vi "Collapse Patterns SLM.vi"(2 "Action":u16(ring) items=["Read", "Initialize"], 7 "collapsed mode array":dbl[][](array[numeric]), 9 "Vortex":dbl[][](array[numeric]), 11 "Top hat":dbl[][](array[numeric])) -> (8 "collapsed patterns":dbl[][](array[numeric]))   [LabVIEW 2014]
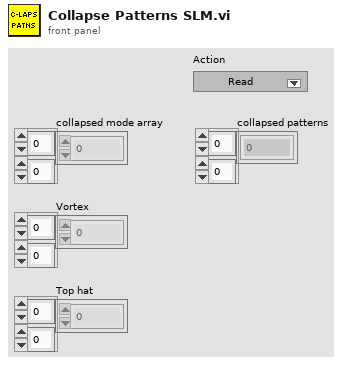
[diagram p1: front panel]
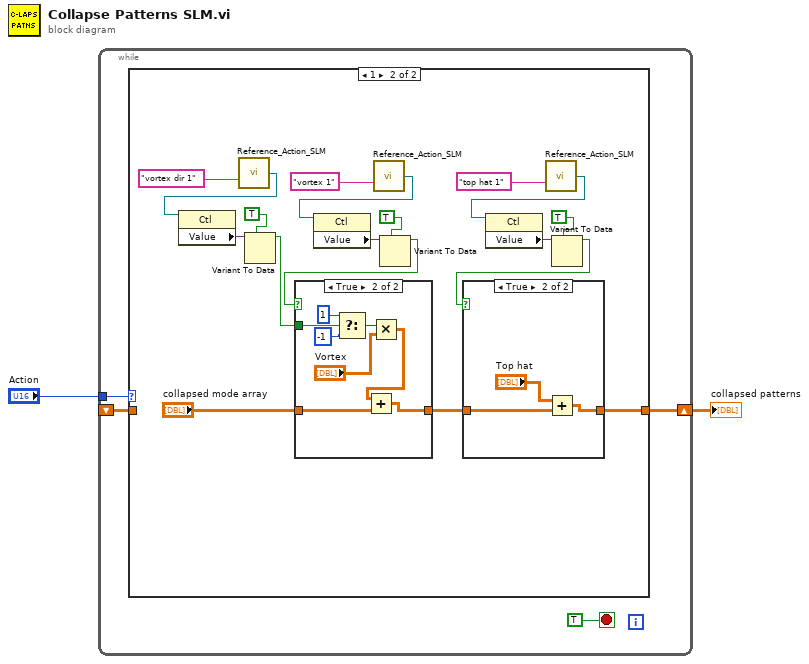
[diagram p0: block diagram]
diagram:
  n1 = while {
    shift-right: [w3] -> w1
    shift-left: _ -> [w4]
    tunnel: "Action" -> [w5]
    stop <- TRUE stop-if-true
    n2 = case shown="1" w5 {
      tunnel: w4 -> [w7 _]
      tunnel: [w7 w14] -> w3
      frame 0, Default {
      }
      frame 1 {
        n3 = call "Reference_Action_SLM.vi"("Control Name"="vortex dir 1") -> ("Ref OUT"=w9:refnum<vi>)  [unwired: 12 in, 2 out]
        n4 = property class="Ctl"(reference=w9) -> ("Value"=w11:variant)  [unwired: 1 in, 2 out]
        n5 = Variant To Data(type=TRUE, Variant=w11) -> (data=w8:bool)  [unwired: 1 in, 1 out]
        n6 = call "Reference_Action_SLM.vi"("Control Name"="vortex 1") -> ("Ref OUT"=w24:refnum<vi>)  [unwired: 12 in, 2 out]
        n7 = property class="Ctl"(reference=w24) -> ("Value"=w23:variant)  [unwired: 1 in, 2 out]
        n8 = Variant To Data(type=TRUE, Variant=w23) -> (data=w21:bool)  [unwired: 1 in, 1 out]
        n9 = case shown="True" w21 {
          tunnel: "collapsed mode array" -> [w30 w38]
          tunnel: [w30 w37] -> w15
          tunnel: w8 -> [_ w31]
          frame False {
          }
          frame True {
            n10 = Select(t=1, s=w31, f=-1) -> (s? t:f=w34:i32)
            n11 = Multiply(x=w34, y="Vortex") -> (x*y=w32:dbl[][])
            n12 = Add(x=w32, y=w38) -> (x+y=w37:dbl[][])
          }
        }
        n13 = call "Reference_Action_SLM.vi"("Control Name"="top hat 1") -> ("Ref OUT"=w19:refnum<vi>)  [unwired: 12 in, 2 out]
        n14 = property class="Ctl"(reference=w19) -> ("Value"=w18:variant)  [unwired: 1 in, 2 out]
        n15 = Variant To Data(type=TRUE, Variant=w18) -> (data=w16:bool)  [unwired: 1 in, 1 out]
        n16 = case shown="True" w16 {
          tunnel: w15 -> [w26 w29]
          tunnel: [w26 w28] -> w14
          frame False {
          }
          frame True {
            n17 = Add(x="Top hat", y=w29) -> (x+y=w28:dbl[][])
          }
        }
      }
    }
  }
  "collapsed patterns" <- w1
